vi "Configure Hardware.vi"(8 "error in (no error)":errorcluster, 11 "Hardware Resources in":T1) -> (0 "error out":errorcluster, 3 "Hardware Resources out":T1)   [LabVIEW 2016, in "Acquisition.lvlib"]
doc: "Configure the hardware."
uses:
  Acquisition.lvlib
  Hardware Configuration.ctl
  <vilib>/DAQmx/create/channels.llb/DAQmx Create Channel (AI-Voltage-Basic).vi
  <vilib>/DAQmx/create/scale.llb/DAQmx Create Scale (Linear).vi
  <vilib>/DAQmx/configure/timing.llb/DAQmx Timing (Sample Clock).vi
  <resource>/objmgr/daqmx.rc
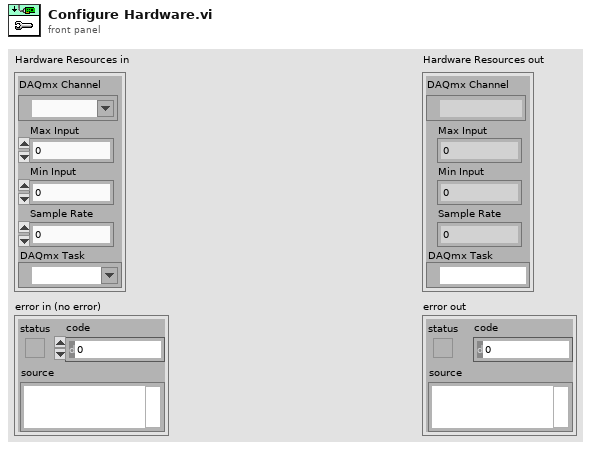
[diagram p1: front panel]
types:
  T1 = typedef "Acquisition.lvlib/Hardware Configuration.ctl" = cluster{"DAQmx Channel":tag, "Max Input":dbl, "Min Input":dbl, "Sample Rate":dbl, "DAQmx Task":refnum<k21>}
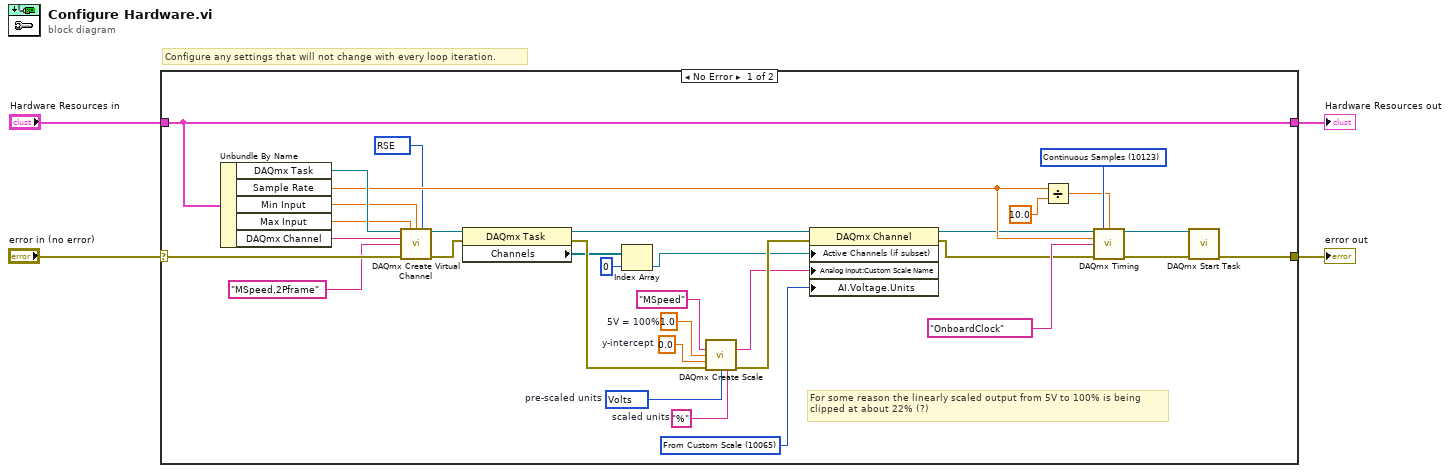
[diagram p0: block diagram]
diagram:
  # "Configure any settings that will not change with every loop iteration."
  n1 = case shown="No Error" "error in (no error)" {
    selector: "error in (no error)" -> [w33 w38]
    tunnel: [w25 w38] -> w3
    tunnel: "Hardware Resources in" -> [w32 w39]
    tunnel: [w32 w39] -> w1
    frame No Error {
      w7 = "%"  # scaled units
      w8 = 10348 items=["Volts"=10348, "Amps"=10342, "Deg F"=10144, "Deg C"=10143, "Deg R"=10145, "Kelvins"=10325, "Strain"=10299, "Ohms"=10384, "Hz"=10373, "Seconds"=10364, "Meters"=10219, "Inches"=10379, "Degrees"=10146, "Radians"=10273, "Ticks"=10304, "g"=10186, "m/s^2"=12470, "m/s"=15959, "in/s"=15960, "Pascals"=10081, "Newtons"=15875, "Pounds"=15876, "kgf"=15877, "psi"=15879, "bar"=15880, "Nm"=15881, "oz-in"=15882, "lb-in"=15883, "lb-ft"=15884, "Volts/Volt"=15896, "mVolts/Volt"=15897, "From TEDS"=12516]  # pre-scaled units
      w6 = 10065 items=["Volts"=10348, "From Custom Scale"=10065, "From TEDS"=12516] ("AI.Voltage.Units")
      w12 = 0.0  # y-intercept
      w13 = 1.0  # 5V = 100%
      w23 = 10083 items=["Default"=-1, "RSE"=10083, "NRSE"=10078, "Differential"=10106, "Pseudodifferential"=12529] ("input terminal configuration")
      w31 = 10123 items=["Finite Samples"=10178, "Continuous Samples"=10123, "Hardware Timed Single Point"=12522] ("sample mode")
      # "For some reason the linearly scaled output from 5V to 100% is being\nclipped at about 22% (?)"
      n2 = Unbundle By Name(w32) -> ("DAQmx Task"=w37:refnum<k21>, "Sample Rate"=w30:dbl, "Min Input"=w34:dbl, "Max Input"=w35:dbl, "DAQmx Channel"=w36:tag)
      n3 = call-poly <vilib>:"DAQmx Create Virtual Channel.vi"("task in"=w37, "maximum value"=w35, "minimum value"=w34, "input terminal configuration"=w23, "physical channels"=w36, "name to assign"="MSpeed,2Pframe", "error in"=w33) -> ("task out"=w22:refnum<k21>, "error out"=w21:errorcluster)  [unwired: 7 in]
      n4 = property class="DAQmx Task"(reference=w22, error in=w21) -> (reference out=w17:refnum<k21>, error out=w16:errorcluster, "Channels"=w11:refnum<k21>[])
      n5 = Index Array(array=w11, index=0) -> (element=w10:refnum<k21>)
      n6 = call-poly <vilib>:"DAQmx Create Scale.vi"("name"="MSpeed", "slope"=w13, "y-intercept"=w12, "error in"=w16, "pre-scaled units"=w8, "scaled units"=w7) -> ("scale out"=w18:tag, "error out"=w19:errorcluster)  [unwired: 8 in]
      n7 = property class="DAQmx Channel"(reference=w17, error in=w19, "Active Channels (if subset)"=w10, "Analog Input:Custom Scale Name"=w18, "AI.Voltage.Units"=w6) -> (reference out=w14:refnum<k21>, error out=w15:errorcluster)
      n8 = Divide(x=w30, y=10.0) -> (x/y=w28:dbl)
      n9 = call-poly <vilib>:"DAQmx Timing.vi"("task/channels in"=w14, "sample mode"=w31, "samples per channel"=w28, "rate"=w30, "source"=tag "OnboardClock", "error in"=w15) -> ("task out"=w26:refnum<k21>, "error out"=w27:errorcluster)  [unwired: 8 in]
      n10 = call <vilib>:"DAQmx Start Task.vi"("task/channels in"=w26, "error in"=w27) -> ("error out"=w25:errorcluster)  [unwired: 12 in, 1 out]
    }
    frame Error {
    }
  }
  "Hardware Resources out" <- w1
  "error out" <- w3
